vi "limit.vi"(1 "Lower_Limit":dbl, 2 "Upper_Limit":dbl, 5 "Input":dbl) -> (0 "Output":dbl)   [LabVIEW 2023]
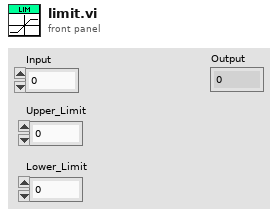
[diagram p1: front panel]
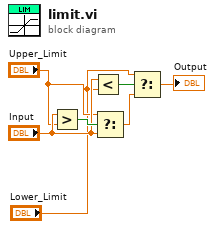
[diagram p0: block diagram]
diagram:
  n1 = Greater?(x="Input", y="Upper_Limit") -> (0:w6:bool)
  n2 = Less?(x="Input", y="Lower_Limit") -> (x < y?=w5:bool)
  n3 = Select(t="Upper_Limit", s=w6, f="Input") -> (s? t:f=w4:dbl)
  n4 = Select(t="Lower_Limit", s=w5, f=w4) -> (s? t:f=→"Output":dbl)
